vi "MH_T2Interface.vi"(8 "error in (no error)":errorcluster caption="entrée d'erreur (pas d'erreur)", 10 "DataProcessQ":refnum<queue>, 11 "Device In":refnum<class "MultiHarp150.lvclass">) -> (0 "error out":errorcluster caption="sortie d'erreur")   [LabVIEW 2019, in "MultiHarp150.lvclass"]
uses:
  MultiHarp150.lvclass
  <userlib>/MultiHarp150/T2Lib/MH_T2QMessage.ctl
  MultiHarp150.lvclass/MultiHarp150.ctl
panel:
  in  "stop":bool
  out "Init Program":bool
  in  "OpCount":i32
  in  "CorrChannels":i32[][](array[numeric])
  out "NextTimeCh":i32
  out "ChIndex":i32[](array[numeric])
  in  "WinSize(bins)":u64
  in  "RefIndex":i32
  in  "ChCount":i32
  out "CorrData":u64[][](array[numeric])
  in  "Datasize":i32
  in  "Max T(s)":i32=1 min=1 max=10000 step=1
  in  "Show Avg":bool
  in  "Avg Val":i32=1 min=1 max=10000 step=1
  in  "Ch":enum16{"Ch1", "Ch2", "Ch3", "Ch4"}(ring)
  out "Graph":cluster{dbl, dbl, i32[]}(graph)
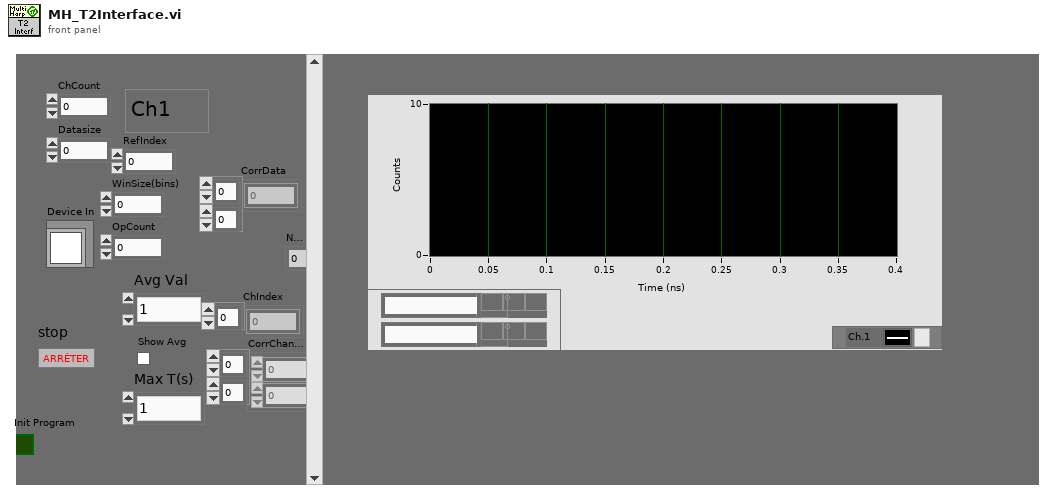
[diagram p1: front panel]
types:
  T1 = typedef "MH_T2QMessage.ctl" = cluster{"Message":string, "buffer":u32[], "Code":i32, "nactual":i32}
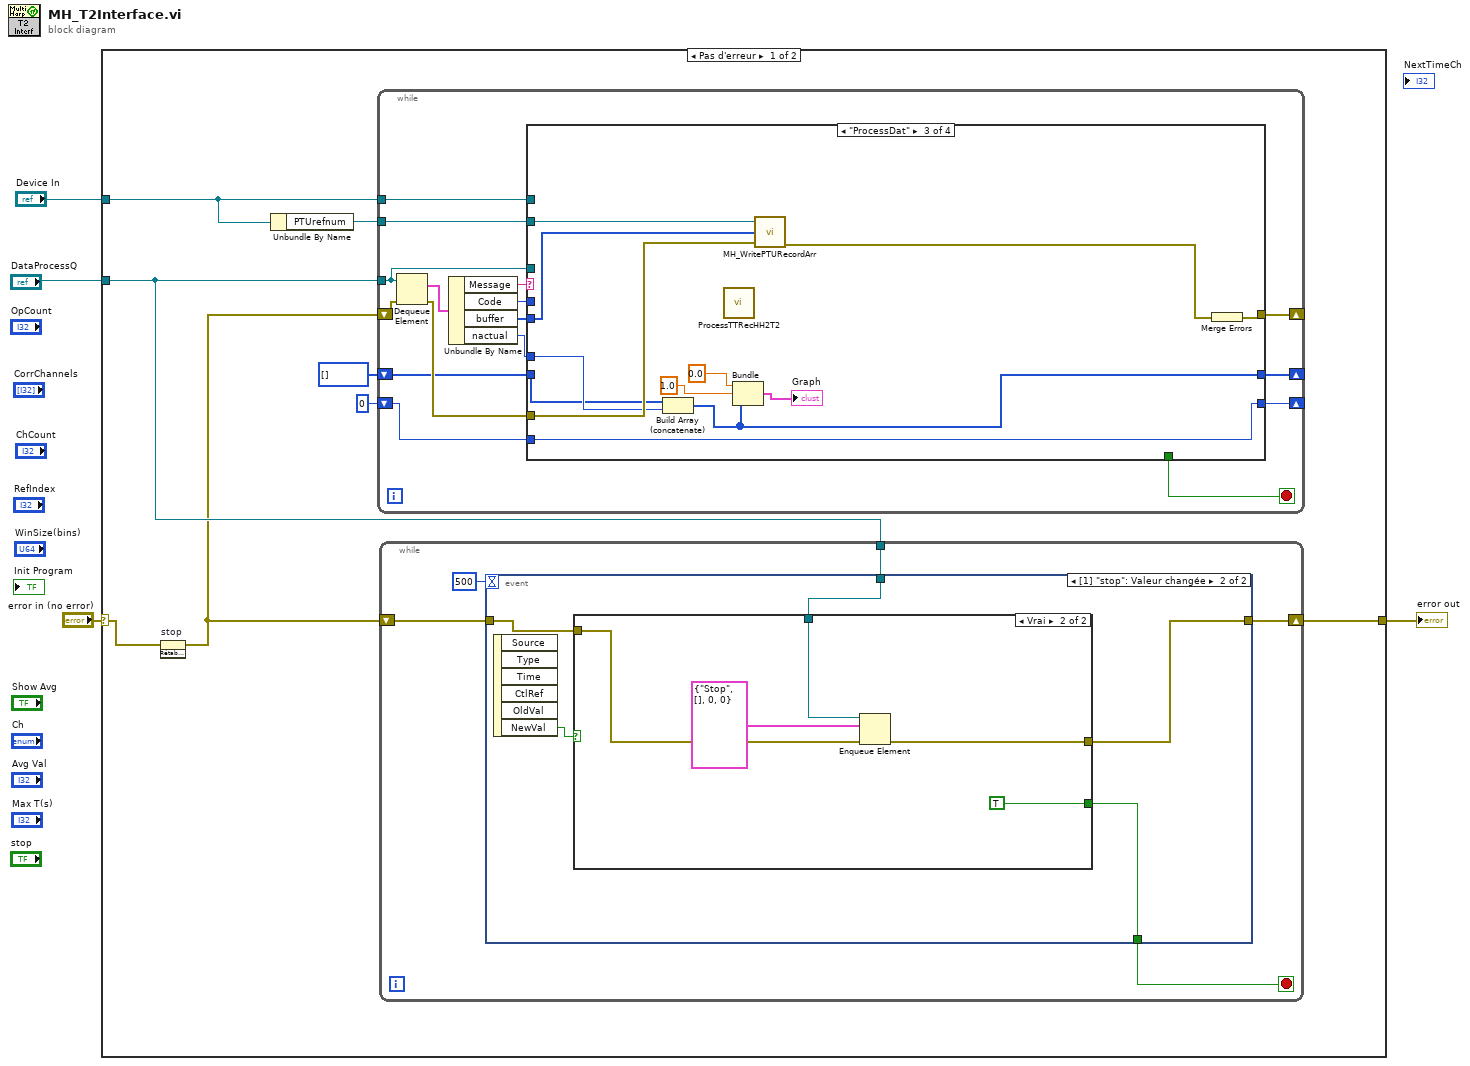
[diagram p0: block diagram]
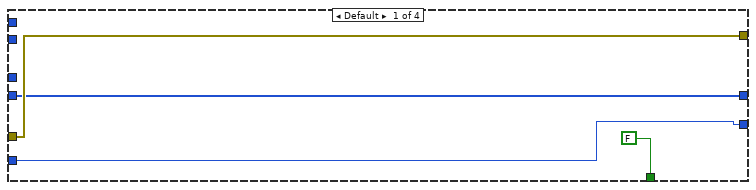
[diagram p2: hidden frame]
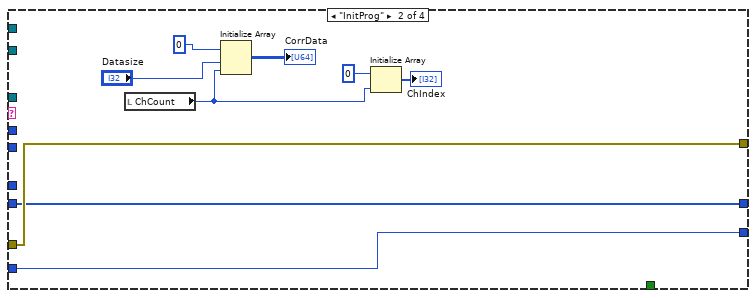
[diagram p3: hidden frame]
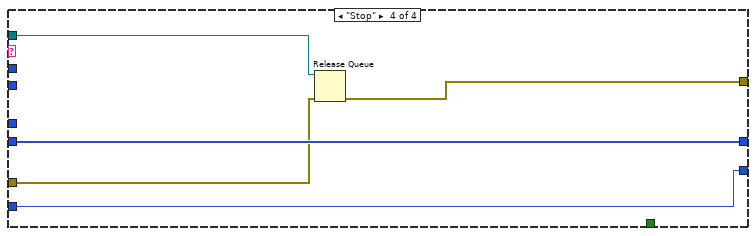
[diagram p4: hidden frame]
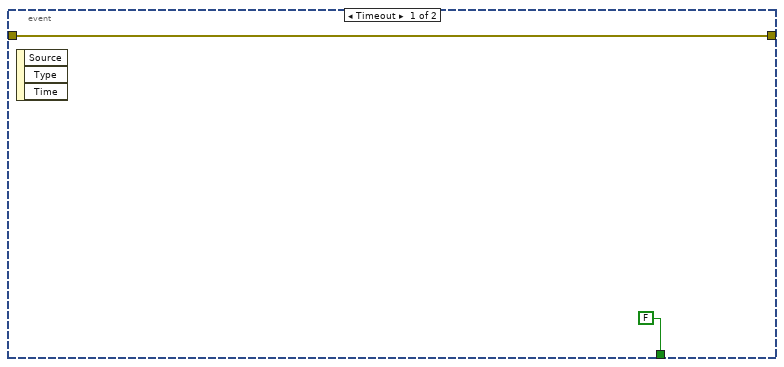
[diagram p5: hidden frame]
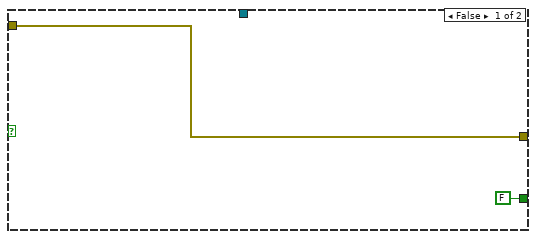
[diagram p6: hidden frame]
diagram:
  n1 = case shown="Pas d'erreur" "error in (no error)" {
    selector: "error in (no error)" -> [w6 w77]
    tunnel: [w12 w77] -> w4
    tunnel: "DataProcessQ" -> [w7 _]
    tunnel: "Device In" -> [w10 _]
    frame No Error {
      n2 = invoke on="stop" class="Bool (strict)" method="RétablirValParDéfaut"(error in=w6) -> (error out=w5:errorcluster)  [unwired: 2 in, 2 out]
      n3 = Unbundle By Name(w10) -> ("PTUrefnum"=w9:refnum<file>)
      n4 = while {
        tunnel: w7 -> [w13]
        shift-right: [w23] -> _
        shift-left: w5 -> [w28]
        shift-right: [w21] -> _
        shift-left: u64 0 ("oflcorr_out") -> [w20]
        tunnel: w10 -> [w19]
        tunnel: w9 -> [w18]
        shift-right: [w15] -> _
        shift-left: i32[] [] -> [w14]
        stop <- w22 stop-if-true
        n5 = Dequeue Element(queue=w13, error in (no error)=w28) -> (element=w17:T1, error out=w27:errorcluster)  [unwired: 1 in, 2 out]
        n6 = Unbundle By Name(w17) -> ("Message"=w26:string, "Code"=w24:i32, "buffer"=w25:u32[], "nactual"=w16:i32)
        n7 = case shown="\"ProcessDat\"" w26 {
          tunnel: w27 -> [w32 w41 w52 w56]
          tunnel: w25 -> [_ _ w49 _]
          tunnel: w24 -> [_ _ _ _]
          tunnel: [w32 w41 w51 w55] -> w23
          tunnel: [FALSE _ _ _] -> w22
          tunnel: [w30 w40 w50 w57] -> w21
          tunnel: w20 -> [w30 w40 w50 w57]
          tunnel: w19 -> [_ _ _ _]
          tunnel: w18 -> [_ _ w53 _]
          tunnel: w16 -> [_ _ w44 _]
          tunnel: [w29 w33 w43 w58] -> w15
          tunnel: w14 -> [w29 w33 w42 w58]
          tunnel: w13 -> [_ _ _ w54]
          frame Default {
          }
          frame "InitProg" {
            n8 = local read "ChCount"() -> (w36:i32)
            n9 = Initialize Array(u64 0 ("oflcorr_out"), "Datasize", w36) -> (→"CorrData":u64[][])
            n10 = Initialize Array(0 ("RefIndex"), w36) -> (→"ChIndex":i32[])
          }
          frame "ProcessDat" {
            n11 = Build Array (concatenate)(w42, w44) -> (w43:i32[])
            n12 = call <userlib>:"ProcessTTRecHH2T2.vi"() -> ()  [unwired: 6 in, 6 out]
            n13 = Bundle(0.0, 1.0, w43) -> (→"Graph":cluster{dbl, dbl, i32[]})  [unwired: 1 in]
            n14 = call <userlib>:"MH_WritePTURecordArr.vi"("refnum"=w53, "TTTR Records"=w49, "error in"=w52) -> ("error out"=w48:errorcluster)  [unwired: 6 in, 1 out]
            n15 = Merge Errors(w48) -> (w51:errorcluster)
          }
          frame "Stop" {
            n16 = Release Queue(queue=w54, error in (no error)=w56) -> (error out=w55:errorcluster)  [unwired: 1 in, 2 out]
          }
        }
      }
      n17 = while {
        shift-right: [w62] -> w12
        shift-left: w5 -> [w61]
        tunnel: w7 -> [w59]
        stop <- w60 stop-if-true
        n18 = event shown="[1] \"stop\": Valeur changée" {
          selector: _ -> [_ _]
          dyn-events: _ -> [_ _]
          timeout: 500 -> [_ _]
          tunnel: [w65 w67] -> w62
          tunnel: w61 -> [w65 w69]
          tunnel: [FALSE w66] -> w60
          tunnel: w59 -> [_ w68]
          event Timeout {
            n19 = event-data() -> ()  [unwired: 1 in, 3 out]
          }
          event "stop": Value Change {
            n20 = event-data() -> ("NewVal"=w70:bool)  [unwired: 1 in, 5 out]
            n21 = case shown="Vrai" w70 {
              tunnel: w69 -> [w72 w73]
              tunnel: w68 -> [_ w76]
              tunnel: [w72 w73] -> w67
              tunnel: [FALSE TRUE] -> w66
              frame False {
              }
              frame True {
                n22 = Enqueue Element(queue=w76, element=T1 {"Message"="Stop", "buffer"=[], "Code"=0, "nactual"=0} ("élément")) -> ()  [unwired: 2 in, 3 out]
              }
            }
          }
        }
      }
    }
    frame Error {
    }
  }
  "error out" <- w4
